vi "QSM - Stop.vi"(6 "QSM":T1={"Invalid Option"=enum."Ignore", "QSM"=refnum}, 7 "Act? (T)":bool=TRUE, 8 "error in (no error)":errorcluster) -> (0 "error out":errorcluster)   [LabVIEW 2014]
doc: "This enqueues the VI Stop State. This ensures, this is always the last state to run.\n\nDataEtc Copyright (c) 2013"
uses:
  TypeDef/QSM - STYP.ctl
  TypeDef/Invalid Option - STYP.ctl
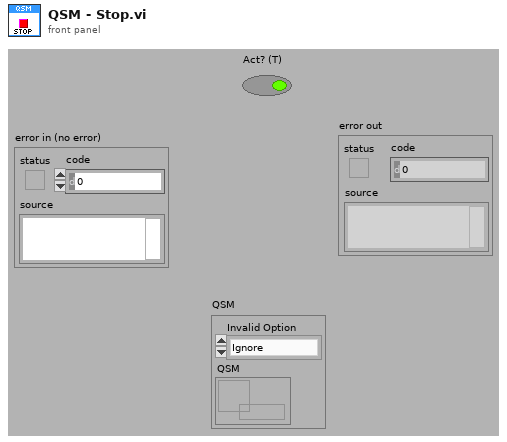
[diagram p1: front panel]
types:
  T1 = typedef "QSM - STYP.ctl" = cluster{"Invalid Option":T2, "QSM":refnum<queue>}
  T2 = typedef "Invalid Option - STYP.ctl" = enum16{"Dialog", "Error", "Ignore"}
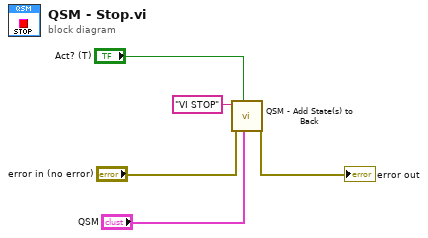
[diagram p0: block diagram]
diagram:
  n1 = call "QSM - Add State(s) to Back.vi"("QSM"="QSM", "Act? (T)"="Act? (T)", "error in (no error)"="error in (no error)", "State(s)"="VI STOP") -> ("error out"=→"error out":errorcluster)  [unwired: 7 out]
